vi "check_start_conditions.vi"(4 "FIFO overflow?":bool, 6 "stop at FIFO overflow?":bool, 7 "converter box version":i16=2 min=1 max=2, 9 "FPGA Scan Counters":T1={"Current part of waveform"=2, "Current waveform"=0} {"Current part of waveform" items=["Imaging", "Settling", "Resting"]}, 10 "wait for trigger?":bool, 11 "Scan":bool) -> (1 "Scanning?":bool, 2 "acquire?":bool)   [LabVIEW 2010]
uses:
  FPGA_Typedefs/FPGA Scan Counters.ctl
  <vilib>/eio/EIONode/EIONode.xnode
  <vilib>/rvi/eio/nirviEIOImplementation/nirviEIOImplementation.xnode
  <vilib>/rvi/eio/common/nirviEmuClasses.ctl
  <vilib>/rvi/eio/common/nirviEmuTemplateMethod_noerrors.vi
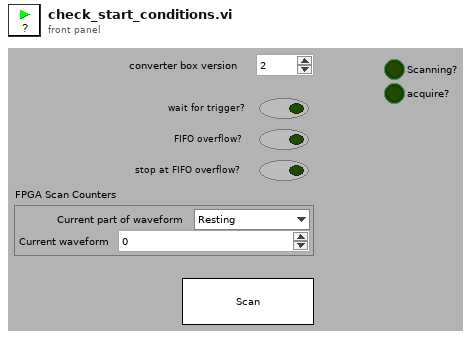
[diagram p1: front panel]
types:
  T1 = typedef "FPGA Scan Counters.ctl" = cluster{"Current part of waveform":u8, "Current waveform":u16}
  T2 = typedef "nirviEmuClasses.ctl" = enum16{"IO Read", "IO Write", "Method", "Property Read", "Property Write"}
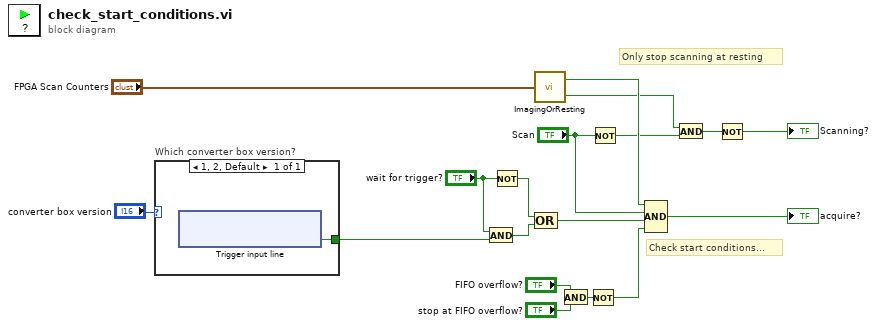
[diagram p0: block diagram]
diagram:
  # "Only stop scanning at resting"
  # "Check start conditions..."
  n1 = case "Which converter box version?" shown="1, 2, Default" "converter box version" {
    tunnel: [w19] -> w17
    frame 1, 2, Default {
      n2 = xnode "Trigger input line"() -> ("Connector0/DIO34"=w19:bool)  [unwired: 1 in, 1 out]
    }
  }
  n3 = And(x="wait for trigger?", y=w17) -> (x .and. y?=w15:bool)
  n4 = Not(x="wait for trigger?") -> (.not. x?=w18:bool)
  n5 = call "ImagingOrResting.vi"("Scan counters"="FPGA Scan Counters") -> ("Currently at resting part?"=w3:bool, "Currently at imaging part?"=w7:bool)
  n6 = Compound Arithmetic op=OR(w18, w15) -> (w10:bool)
  n7 = And(x="FIFO overflow?", y="stop at FIFO overflow?") -> (x .and. y?=w12:bool)
  n8 = Not(x=w12) -> (.not. x?=w9:bool)
  n9 = Not(x="Scan") -> (.not. x?=w4:bool)
  n10 = Compound Arithmetic op=AND(w7, "Scan", w10, w9) -> (→"acquire?":bool)
  n11 = And(x=w3, y=w4) -> (x .and. y?=w2:bool)
  n12 = Not(x=w2) -> (.not. x?=→"Scanning?":bool)
